vi "АиР_auto.vi"() -> ()   [LabVIEW 2016]
uses:
  <vilib>/Analysis/5stat.llb/RMS (DBL).vi
  <vilib>/Instr/_visa.llb/VISA Configure Serial Port (Instr).vi
  <vilib>/Analysis/NI_AALPro.lvlib
panel:
  out "I,A 2":dbl
  out "R_ end":dbl
  out "Error":dbl
  in  "I, A":dbl
  out "R_v":dbl
  out "R_h":dbl
  out "R":dbl
  out "U, V":dbl
  in  "Voltmeter":refnum<visa-resource-name>
  out "I,A":dbl
  in  "Relay":refnum<visa-resource-name>
  in  "Source":refnum<visa-resource-name>
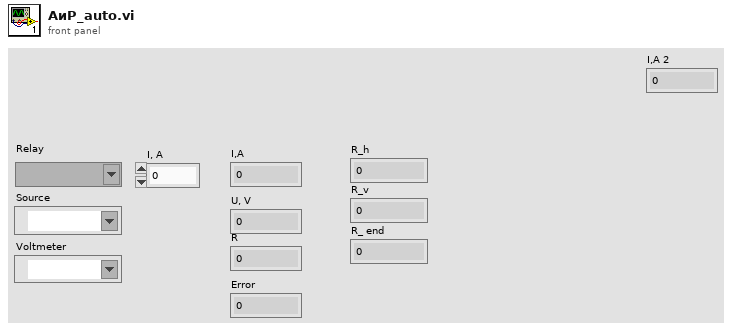
[diagram p1: front panel]
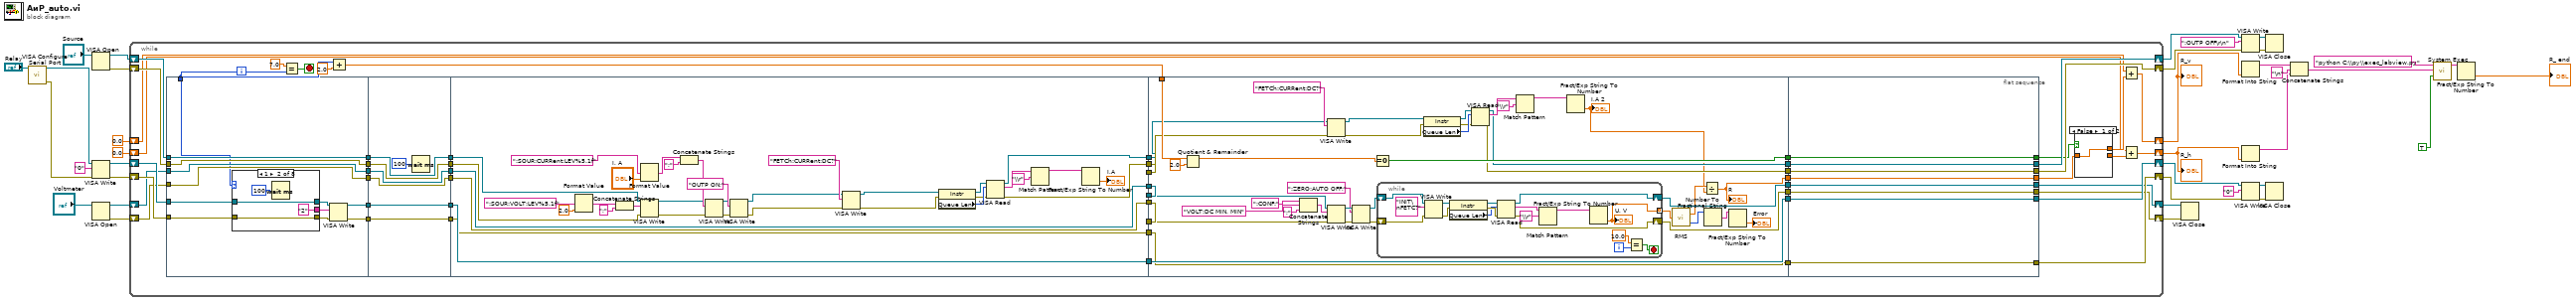
[diagram p0: block diagram]
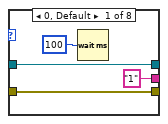
[diagram p3: hidden frame]
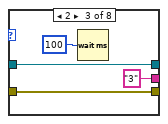
[diagram p4: hidden frame]
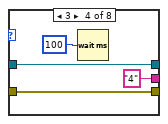
[diagram p5: hidden frame]
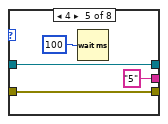
[diagram p6: hidden frame]
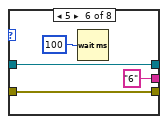
[diagram p7: hidden frame]
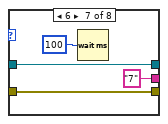
[diagram p8: hidden frame]
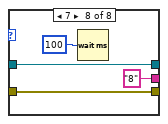
[diagram p9: hidden frame]
diagram:
  n1 = call-poly "VISA Configure Serial Port"("VISA resource name"="Relay") -> ("VISA resource name out"=w17:refnum<visa-resource-name>, "error out"=w16:errorcluster)  [unwired: 13 in]
  n2 = VISA Open(VISA resource name="Source") -> (VISA resource name=w29:refnum<visa-resource-name>, error out=w28:errorcluster)  [unwired: 4 in]
  n3 = VISA Write(VISA resource name=w17, write buffer="0", error in (no error)=w16) -> (VISA resource name out=w19:refnum<visa-resource-name>, error out=w18:errorcluster)  [unwired: 1 out]
  n4 = VISA Open(VISA resource name="Voltmeter") -> (VISA resource name=w26:refnum<visa-resource-name>, error out=w25:errorcluster)  [unwired: 4 in]
  n5 = while {
    shift-right: [w84] -> w15
    shift-left: w19 -> [w87]
    shift-right: [w85] -> w14
    shift-left: w18 -> [w86]
    shift-right: [w83] -> w31
    shift-left: w29 -> [w81]
    shift-right: [w82] -> w30
    shift-left: w28 -> [w80]
    shift-right: [w77] -> w24
    shift-left: w26 -> [w79]
    shift-right: [w76] -> w23
    shift-left: w25 -> [w78]
    shift-right: [w53] -> w4
    shift-left: 0.0 -> [w52]
    shift-right: [w51] -> w5
    shift-left: 0.0 -> [w55]
    i -> [w60]
    stop <- w62 stop-if-true
    n6 = flat-sequence {
      tunnel: [w95] -> w75
      tunnel: [w96] -> w73
      tunnel: [w92] -> w71
      tunnel: [w91] -> w69
      tunnel: [w99] -> w67
      tunnel: [w98] -> w65
      tunnel: w60 -> [w90]
      tunnel: w87 -> [w94]
      tunnel: w86 -> [w93]
      tunnel: w81 -> [w92]
      tunnel: w80 -> [w91]
      tunnel: w79 -> [w99]
      tunnel: w78 -> [w98]
      tunnel: w75 -> [w140]
      tunnel: [w140] -> w74
      tunnel: w73 -> [w139]
      tunnel: [w139] -> w72
      tunnel: w71 -> [w138]
      tunnel: [w138] -> w70
      tunnel: w69 -> [w137]
      tunnel: [w137] -> w68
      tunnel: w67 -> [w136]
      tunnel: [w136] -> w66
      tunnel: w65 -> [w135]
      tunnel: [w135] -> w64
      tunnel: w74 -> [w145]
      tunnel: w72 -> [w146]
      tunnel: [w166] -> w44
      tunnel: [w165] -> w43
      tunnel: w70 -> [w152]
      tunnel: w68 -> [w151]
      tunnel: [w164] -> w42
      tunnel: w66 -> [w164]
      tunnel: w64 -> [w163]
      tunnel: [w163] -> w41
      tunnel: [w146] -> w40
      tunnel: [w145] -> w39
      tunnel: w44 -> [w179]
      tunnel: w43 -> [w180]
      tunnel: w42 -> [w203]
      tunnel: w41 -> [w202]
      tunnel: w59 -> [w201]
      tunnel: [w191] -> w50
      tunnel: [w178] -> w49
      tunnel: [w205] -> w48
      tunnel: [w204] -> w47
      tunnel: [w198] -> w46
      tunnel: [w197] -> w45
      tunnel: w40 -> [w191]
      tunnel: w39 -> [w190]
      tunnel: [w190] -> w38
      tunnel: [w177] -> w37
      tunnel: [w232] -> w57
      tunnel: [w233] -> w58
      tunnel: [w234] -> w76
      tunnel: [w235] -> w77
      tunnel: [w236] -> w82
      tunnel: [w237] -> w83
      tunnel: [w238] -> w84
      tunnel: [w239] -> w85
      tunnel: w50 -> [w238]
      tunnel: w49 -> [w237]
      tunnel: w48 -> [w235]
      tunnel: w47 -> [w234]
      tunnel: w46 -> [w233]
      tunnel: w45 -> [w232]
      tunnel: w38 -> [w239]
      tunnel: w37 -> [w236]
      frame #0 {
        n7 = case shown="1" w90 {
          tunnel: ["1" "2" "3" "4" "5" "6" "7" "8"] -> w97
          tunnel: [w103 w107 w111 w115 w119 w123 w127 w131] -> w101
          tunnel: w94 -> [w103 w107 w111 w115 w119 w123 w127 w131]
          tunnel: [w102 w106 w110 w114 w118 w122 w126 w130] -> w100
          tunnel: w93 -> [w102 w106 w110 w114 w118 w122 w126 w130]
          frame 0, Default {
            n8 = Wait (ms)(milliseconds to wait=u32 100) -> ()  [unwired: 1 out]
          }
          frame 1 {
            n9 = Wait (ms)(milliseconds to wait=u32 100) -> ()  [unwired: 1 out]
          }
          frame 2 {
            n10 = Wait (ms)(milliseconds to wait=u32 100) -> ()  [unwired: 1 out]
          }
          frame 3 {
            n11 = Wait (ms)(milliseconds to wait=u32 100) -> ()  [unwired: 1 out]
          }
          frame 4 {
            n12 = Wait (ms)(milliseconds to wait=u32 100) -> ()  [unwired: 1 out]
          }
          frame 5 {
            n13 = Wait (ms)(milliseconds to wait=u32 100) -> ()  [unwired: 1 out]
          }
          frame 6 {
            n14 = Wait (ms)(milliseconds to wait=u32 100) -> ()  [unwired: 1 out]
          }
          frame 7 {
            n15 = Wait (ms)(milliseconds to wait=u32 100) -> ()  [unwired: 1 out]
          }
        }
        n16 = VISA Write(VISA resource name=w101, write buffer=w97, error in (no error)=w100) -> (VISA resource name out=w96:refnum<visa-resource-name>, error out=w95:errorcluster)  [unwired: 1 out]
      }
      frame #1 {
        n17 = Wait (ms)(milliseconds to wait=u32 100) -> ()  [unwired: 1 out]
      }
      frame #2 {
        n18 = Format Value(format string=":SOUR:VOLT:LEV%5.1f" ("write buffer"), value (0)=2.0) -> (output string=w156:string)  [unwired: 1 in]
        n19 = Concatenate Strings(w156, ";" ("string")) -> (w154:string)
        n20 = Format Value(format string=":SOUR:CURRent:LEV%5.1f" ("write buffer"), value (0)="I, A") -> (output string=w162:string)  [unwired: 1 in]
        n21 = VISA Write(VISA resource name=w152, write buffer=w154, error in (no error)=w151) -> (VISA resource name out=w150:refnum<visa-resource-name>, error out=w149:errorcluster)  [unwired: 1 out]
        n22 = Concatenate Strings(w162, ";" ("string")) -> (w160:string)
        n23 = VISA Write(VISA resource name=w150, write buffer=w160, error in (no error)=w149) -> (VISA resource name out=w159:refnum<visa-resource-name>, error out=w158:errorcluster)  [unwired: 1 out]
        n24 = VISA Write(VISA resource name=w159, write buffer="OUTP ON;", error in (no error)=w158) -> (VISA resource name out=w144:refnum<visa-resource-name>, error out=w143:errorcluster)  [unwired: 1 out]
        n25 = VISA Write(VISA resource name=w144, write buffer="FETCh:CURRent:DC?", error in (no error)=w143) -> (VISA resource name out=w142:refnum<visa-resource-name>, error out=w141:errorcluster)  [unwired: 1 out]
        n26 = property class="Instr"(reference=w142, error in=w141) -> (reference out=w174:refnum<visa-resource-name>, error out=w173:errorcluster, "Queue Len"=w175:u32)
        n27 = VISA Read(VISA resource name=w174, byte count=w175, error in (no error)=w173) -> (VISA resource name out=w166:refnum<visa-resource-name>, read buffer=w169:string, error out=w165:errorcluster)  [unwired: 1 out]
        n28 = Match Pattern(string=w169, regular expression="\\r") -> (before substring=w167:string)  [unwired: 1 in, 3 out]
        n29 = Fract/Exp String To Number(string=w167) -> (number=→"I,A":dbl)  [unwired: 3 in, 1 out]
      }
      frame #3 {
        n30 = Quotient & Remainder(x=w201, y=2.0) -> (x-y*floor(x/y)=w199:dbl)  [unwired: 1 out]
        n31 = Concatenate Strings(":CONF:" ("string (\"\")"), "VOLT:DC MIN, MIN" ("format string"), ";" ("string")) -> (w211:string)
        n32 = VISA Write(VISA resource name=w179, write buffer="FETCh:CURRent:DC?", error in (no error)=w180) -> (VISA resource name out=w182:refnum<visa-resource-name>, error out=w181:errorcluster)  [unwired: 1 out]
        n33 = VISA Write(VISA resource name=w203, write buffer=w211, error in (no error)=w202) -> (VISA resource name out=w210:refnum<visa-resource-name>, error out=w209:errorcluster)  [unwired: 1 out]
        n34 = VISA Write(VISA resource name=w210, write buffer=":ZERO:AUTO OFF;", error in (no error)=w209) -> (VISA resource name out=w207:refnum<visa-resource-name>, error out=w206:errorcluster)  [unwired: 1 out]
        n35 = Equal To 0?(x=w199) -> (x = 0?=w198:bool)
        n36 = while {
          shift-right: [w224] -> w205
          shift-left: w207 -> [w220]
          shift-right: [w223] -> w204
          shift-left: w206 -> [w219]
          tunnel: [w218] -> w196 mode=indexing
          i -> [w215]
          stop <- w217 stop-if-true
          n37 = VISA Write(VISA resource name=w220, write buffer="INIT\nFETC?", error in (no error)=w219) -> (VISA resource name out=w221:refnum<visa-resource-name>, error out=w222:errorcluster)  [unwired: 1 out]
          n38 = property class="Instr"(reference=w221, error in=w222) -> (reference out=w230:refnum<visa-resource-name>, error out=w229:errorcluster, "Queue Len"=w228:u32)
          n39 = VISA Read(VISA resource name=w230, byte count=w228, error in (no error)=w229) -> (VISA resource name out=w224:refnum<visa-resource-name>, read buffer=w226:string, error out=w223:errorcluster)  [unwired: 1 out]
          n40 = Match Pattern(string=w226, regular expression="\\r") -> (before substring=w225:string)  [unwired: 1 in, 3 out]
          n41 = Fract/Exp String To Number(string=w225) -> (number=w218:dbl)  [unwired: 3 in, 1 out]
          "U, V" <- w218
          n42 = Equal?(x=10.0, y=w215) -> (x = y?=w217:bool)
        }
        n43 = property class="Instr"(reference=w182, error in=w181) -> (reference out=w188:refnum<visa-resource-name>, error out=w187:errorcluster, "Queue Len"=w189:u32)
        n44 = VISA Read(VISA resource name=w188, byte count=w189, error in (no error)=w187) -> (VISA resource name out=w178:refnum<visa-resource-name>, read buffer=w185:string, error out=w177:errorcluster)  [unwired: 1 out]
        n45 = Match Pattern(string=w185, regular expression="\\r") -> (before substring=w183:string)  [unwired: 1 in, 3 out]
        n46 = Fract/Exp String To Number(string=w183) -> (number=w176:dbl)  [unwired: 3 in, 1 out]
        "I,A 2" <- w176
        n47 = call-poly <vilib>:"RMS.vi"("X"=w196) -> ("rms value"=w195:dbl, "error"=w194:i32)
        n48 = Divide(x=w195, y=w176) -> (x/y=w197:dbl)
        "R" <- w197
        n49 = Number To Fractional String(number=w194) -> (F-format string=w193:string)  [unwired: 3 in]
        n50 = Fract/Exp String To Number(string=w193) -> (number=→"Error":dbl)  [unwired: 3 in, 1 out]
      }
      frame #4 {
      }
    }
    n51 = Equal?(x=7.0, y=w60) -> (x = y?=w62:bool)
    n52 = Add(x=w60, y=2.0) -> (x+y=w59:dbl)
    n53 = case shown="False" w58 {
      tunnel: w57 -> [w88 w89]
      tunnel: [_ w89] -> w56
      tunnel: [w88 _] -> w54
      frame False {
      }
      frame True {
      }
    }
    n54 = Add(x=w55, y=w54) -> (x+y=w51:dbl)
    n55 = Add(x=w52, y=w56) -> (x+y=w53:dbl)
  }
  "R_h" <- w4
  "R_v" <- w5
  n56 = VISA Close(VISA resource name=w24, error in (no error)=w23) -> ()  [unwired: 1 out]
  n57 = VISA Write(VISA resource name=w31, write buffer=":OUTP OFF\r\n", error in (no error)=w30) -> (VISA resource name out=w35:refnum<visa-resource-name>, error out=w34:errorcluster)  [unwired: 1 out]
  n58 = Format Into String(w5) -> (resulting string=w7:string)  [unwired: 3 in, 1 out]
  n59 = Format Into String(w4) -> (resulting string=w6:string)  [unwired: 3 in, 1 out]
  n60 = VISA Write(VISA resource name=w15, write buffer="0", error in (no error)=w14) -> (VISA resource name out=w12:refnum<visa-resource-name>, error out=w11:errorcluster)  [unwired: 1 out]
  n61 = VISA Close(VISA resource name=w35, error in (no error)=w34) -> ()  [unwired: 1 out]
  n62 = VISA Close(VISA resource name=w12, error in (no error)=w11) -> ()  [unwired: 1 out]
  n63 = Concatenate Strings(w7, "\n" ("string"), w6) -> (w8:string)
  n64 = call <vilib>:"System Exec.vi"("run minimized? (F)"=TRUE, "standard input"=w8, "command line"="python C:\\py\\exec_labview.py" ("standard input")) -> ("standard output"=w3:string)  [unwired: 5 in, 3 out]
  n65 = Fract/Exp String To Number(string=w3) -> (number=→"R_ end":dbl)  [unwired: 3 in, 1 out]
